vi "Read Products.vi"(8 "error in (no error)":errorcluster) -> (0 "error out":errorcluster, 3 "Array":T1(array[cluster]))   [LabVIEW 2020, in "Productos.lvlib"]
uses:
  Productos.lvlib
  <vilib>/Utility/sysdir.llb/System Directory Type.ctl
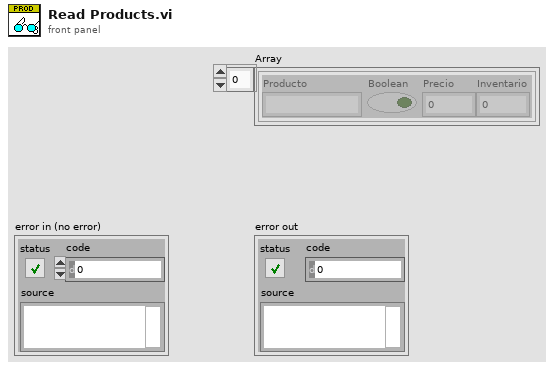
[diagram p1: front panel]
types:
  T1 = cluster{"Producto":string, "Boolean":bool, "Precio":dbl, "Inventario":dbl}[]
  T2 = cluster{"Producto":string, "Boolean":bool, "Precio":dbl, "Precio 2":dbl}[]
  T3 = typedef "System Directory Type.ctl" = i32
  T4 = enum16{"open", "replace", "create", "open or create", "replace or create", "replace or create with confirmation"}
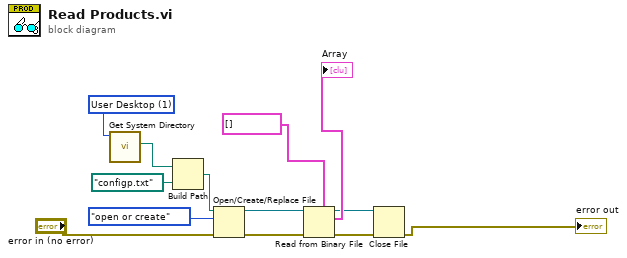
[diagram p0: block diagram]
diagram:
  w8 = T3 1 items=["User Home"=0, "User Desktop"=1, "User Documents"=2, "User Application Data"=3, "User Preferences"=4, "User Temporary"=5, "Public Documents"=6, "Public Application Data"=7, "Public Preferences"=8, "Public Cache"=13, "System Core Libraries"=9, "System Installed Libraries"=10, "Application Files"=11, "Boot Volume Root"=12] ("system directory type")
  n1 = call <vilib>:"Get System Directory.vi"("system directory type"=w8) -> ("system directory"=w7:path)  [unwired: 10 in]
  n2 = Build Path(base path=w7, name or relative path=path "configp.txt") -> (appended path=w5:path)
  n3 = Open/Create/Replace File(file path (use dialog)=w5, error in="error in (no error)", operation (0:open)=T4."open or create") -> (refnum out=w10:refnum<file>, error out=w4:errorcluster)  [unwired: 3 in, 1 out]
  n4 = Read from Binary File(5:T2 [] ("Array"), 8:w4, 11:w10) -> (0:w3:errorcluster, 2:→"Array":T2, 3:w2:refnum<file>)  [unwired: 3 in, 1 out]
  n5 = Close File(refnum=w2, error in=w3) -> (error out=→"error out":errorcluster)  [unwired: 1 out]
